vi "COM_Gauge.vi"() -> ()   [LabVIEW 2013]
uses:
  <vilib>/Instr/_visa.llb/VISA Configure Serial Port (Instr).vi
panel:
  out "Gauge":dbl(knob) scale=1.0..1023.0
  out ".not. x?":bool
  in  "VISA resource name":refnum<visa-resource-name>
  in  "stop":bool
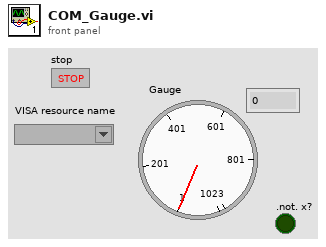
[diagram p1: front panel]
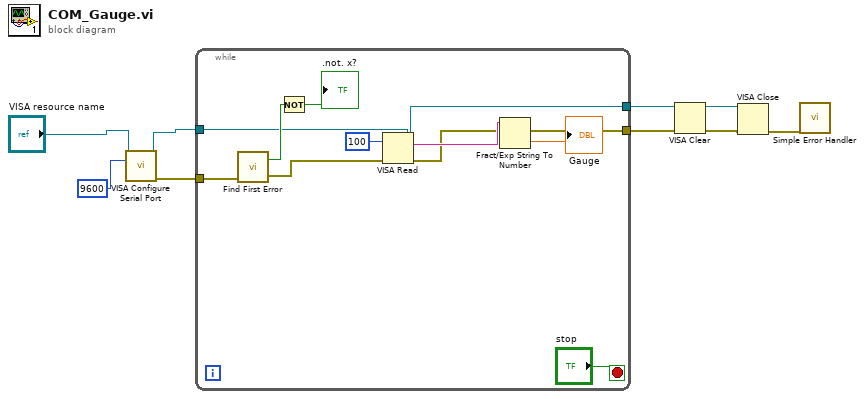
[diagram p0: block diagram]
diagram:
  n1 = call-poly "VISA Configure Serial Port"("VISA resource name"="VISA resource name", "baud rate (9600)"=u32 9600) -> ("VISA resource name out"=w6:refnum<visa-resource-name>, "error out"=w7:errorcluster)  [unwired: 12 in]
  n2 = while {
    tunnel: w7 -> [w19]
    tunnel: w6 -> [w15]
    tunnel: [w11] -> w3
    tunnel: [w10] -> w2
    stop <- "stop" stop-if-true
    n3 = call <vilib>:"Find First Error.vi"("error in (no error)"=w19) -> ("error out"=w16:errorcluster, "error?"=w18:bool)  [unwired: 3 in]
    n4 = Not(x=w18) -> (.not. x?=→".not. x?":bool)
    n5 = VISA Read(VISA resource name=w15, byte count=u32 100, error in (no error)=w16) -> (VISA resource name out=w11:refnum<visa-resource-name>, read buffer=w13:string, error out=w10:errorcluster)  [unwired: 1 out]
    n6 = Fract/Exp String To Number(string=w13) -> (number=→"Gauge":dbl)  [unwired: 3 in, 1 out]
  }
  n7 = VISA Clear(VISA resource name=w3, error in (no error)=w2) -> (VISA resource name out=w5:refnum<visa-resource-name>, error out=w4:errorcluster)
  n8 = VISA Close(VISA resource name=w5, error in (no error)=w4) -> (error out=w1:errorcluster)
  n9 = call <vilib>:"Simple Error Handler.vi"("error in (no error)"=w1) -> ()  [unwired: 4 in, 5 out]
